vi "Read WFChart Refnum.vi"(8 "error in (no error)":errorcluster, 11 "Abstract Sensor in":refnum<class "Abstract Sensor.lvclass">) -> (0 "error out":errorcluster, 2 "WFChart Refnum":refnum<vi>, 3 "Abstract Sensor out":refnum<class "Abstract Sensor.lvclass">)   [LabVIEW 2014, in "Abstract Sensor.lvlib" / "Abstract Sensor.lvclass"]
uses:
  Abstract Sensor.lvclass
  Abstract Sensor.lvclass/Abstract Sensor.ctl
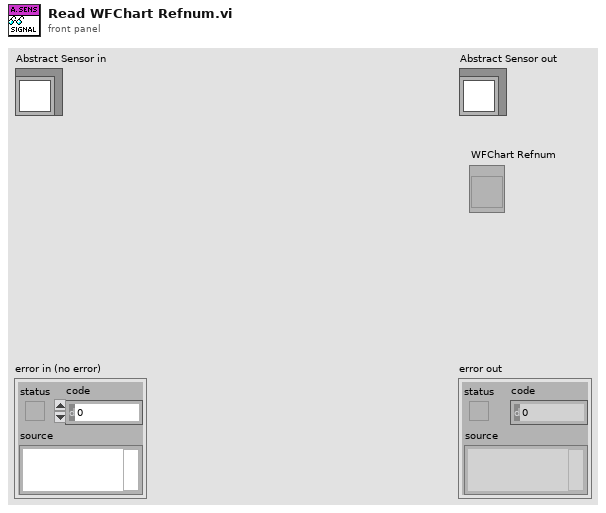
[diagram p1: front panel]
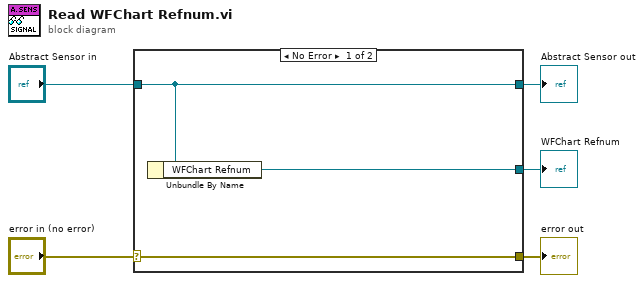
[diagram p0: block diagram]
diagram:
  n1 = case shown="No Error" "error in (no error)" {
    selector: "error in (no error)" -> [w8 w9]
    tunnel: [w8 w9] -> w4
    tunnel: [w7 w10] -> w2
    tunnel: "Abstract Sensor in" -> [w7 w10]
    tunnel: [w6 _] -> w1
    frame No Error {
      n2 = Unbundle By Name(w7) -> ("WFChart Refnum"=w6:refnum<vi>)
    }
    frame Error {
    }
  }
  "error out" <- w4
  "Abstract Sensor out" <- w2
  "WFChart Refnum" <- w1
